vi "PopulateControlsFromCSV.vi"() -> ()   [LabVIEW 2019]
uses:
  <vilib>/Utility/file.llb/Read Delimited Spreadsheet (string).vi
panel:
  out "Label.Text":string
  out "all rows":string[][](array[string])
  in  "Numeric 4":dbl
  in  "Numeric 3":dbl
  in  "Numeric 2":dbl
  in  "Numeric":dbl
  in  "Path":path
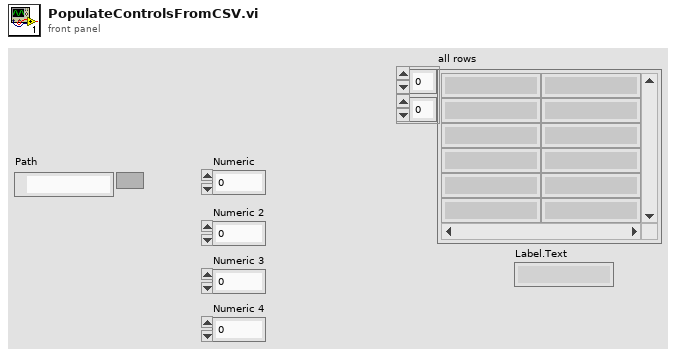
[diagram p1: front panel]
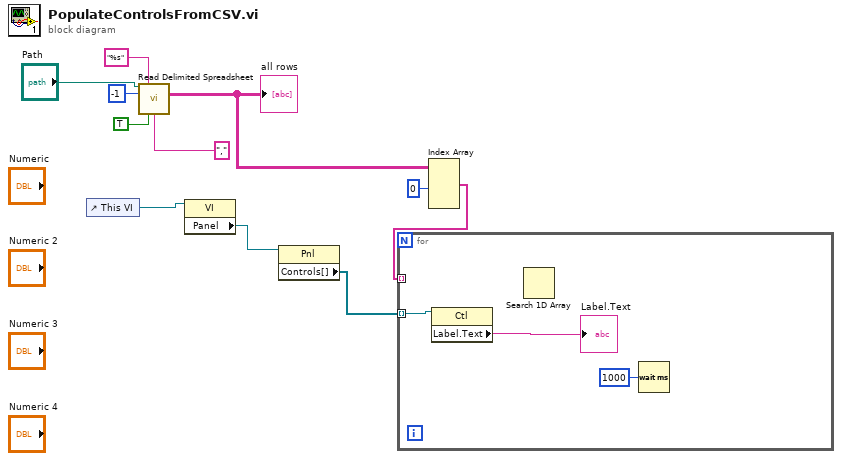
[diagram p0: block diagram]
diagram:
  n1 = control-ref of="This VI"() -> (w8:refnum<vi>)
  n2 = call-poly <vilib>:"Read Delimited Spreadsheet.vi"("file path (dialog if empty)"="Path", "format (%s)"="%s", "number of rows (all:-1)"=-1, "transpose? (F)"=TRUE, "delimiter (\\t)"="," ("delimiter (\\t)")) -> ("all rows"=w3:string[][])  [unwired: 5 in, 5 out]
  "all rows" <- w3
  n3 = property class="VI"(reference=w8) -> ("Panel"=w7:refnum<vi>)  [unwired: 1 in, 2 out]
  n4 = property class="Pnl"(reference=w7) -> ("Controls[]"=w6:refnum<vi>[])  [unwired: 1 in, 2 out]
  n5 = Index Array(array=w3, index (col) #1=0 ("disabled index (col)")) -> (element #1=w2:string[])  [unwired: 3 in, 1 out]
  n6 = for {
    tunnel: w6 -> [w14] mode=indexing
    tunnel: w2 -> [_] mode=indexing
    n7 = property class="Ctl"(reference=w14) -> ("Label.Text"=→"Label.Text":string)  [unwired: 1 in, 2 out]
    n8 = Search 1D Array() -> ()  [unwired: 3 in, 1 out]
    n9 = Wait (ms)(milliseconds to wait=u32 1000) -> ()  [unwired: 1 out]
  }
